vi "HVenable2.vi"(0 "Strings in":string[](array[string])=["C:\\CuspControl\\GPIB and Network\\Cusp\\Dummyfile.txt", "6723"], 1 "Dubs in":dbl[](array[numeric])=[1.0, 20.0]) -> ()   [LabVIEW 2018]
uses:
  <vilib>/DAQmx/write.llb/DAQmx Write (Analog 1D DBL NChan 1Samp).vi
  <vilib>/DAQmx/create/channels.llb/DAQmx Create Channel (AO-Voltage-Basic).vi
  <vilib>/DAQmx/miscellaneous.llb/DAQmx Fill In Error Info.vi
panel:
  in  "Gain (15 V/V)":dbl=15.0
  out "Outvolts":dbl[](array[numeric])
  in  "Enable":bool
  in  "Amplitude (V)":dbl
  in  "subvi":bool=TRUE
  out "error out":errorcluster
  in  "AO2 name":string="6723"
  in  "ao lines":string[](array[string])=["/ao5", "/ao6"]
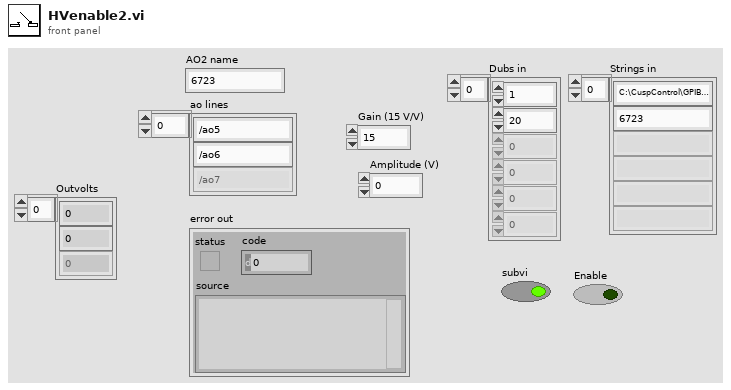
[diagram p1: front panel]
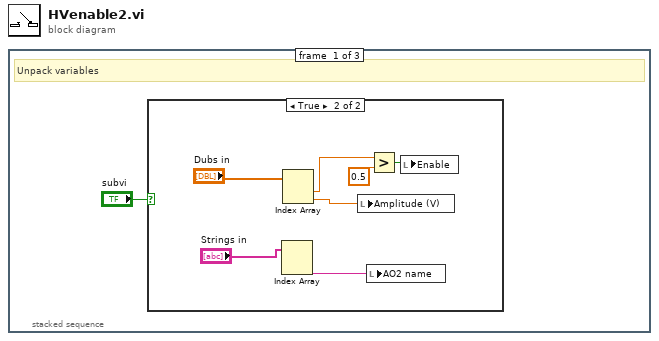
[diagram p0: block diagram]
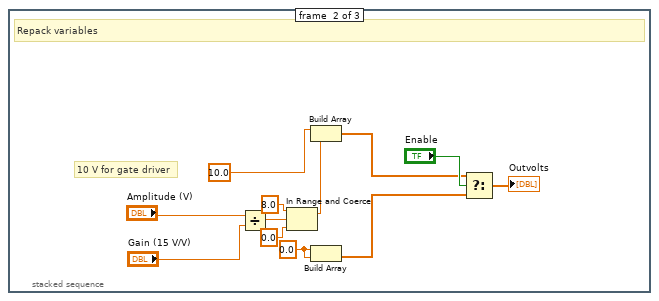
[diagram p3: hidden frame]
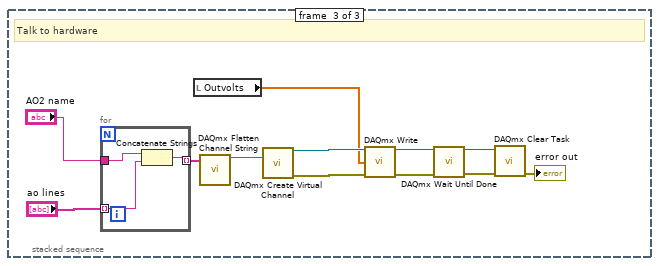
[diagram p4: hidden frame]
diagram:
  n1 = stacked-sequence {
    frame #0 {
      # "Unpack variables"
      n2 = case shown="True" "subvi" {
        frame False {
        }
        frame True {
          n3 = Index Array(array="Strings in") -> (element #2=w6:string)  [unwired: 2 in, 1 out]
          n4 = Index Array(array="Dubs in") -> (element #1=w3:dbl, element #2=w2:dbl)  [unwired: 2 in]
          n5 = local write "Amplitude (V)"(w2) -> ()
          n6 = local write "AO2 name"(w6) -> ()
          n7 = Greater?(x=w3, y=0.5) -> (0:w5:bool)
          n8 = local write "Enable"(w5) -> ()
        }
      }
    }
    frame #1 {
      w19 = 0.0 ("element")
      # "10 V for gate driver"
      # "Repack variables"
      n9 = Divide(x="Amplitude (V)", y="Gain (15 V/V)") -> (x/y=w12:dbl)
      n10 = In Range and Coerce(upper limit=8.0, x=w12, lower limit=0.0) -> (coerced(x)=w11:dbl)  [unwired: 1 out]
      n11 = Build Array(10.0 ("t"), w11) -> (w17:dbl[])
      n12 = Build Array(w19, w19) -> (w16:dbl[])
      n13 = Select(t=w17, s="Enable", f=w16) -> (s? t:f=→"Outvolts":dbl[])
    }
    frame #2 {
      # "Talk to hardware"
      n14 = for {
        tunnel: "ao lines" -> [w33] mode=indexing
        tunnel: "AO2 name" -> [w34]
        tunnel: [w35] -> w23 mode=indexing
        n15 = Concatenate Strings(w34, w33) -> (w35:string)
      }
      n16 = local read "Outvolts"() -> (w21:dbl[])
      n17 = call <vilib>:"DAQmx Flatten Channel String.vi"("names in"=w23) -> ("names out"=w22:string)  [unwired: 13 in, 1 out]
      n18 = call-poly <vilib>:"DAQmx Create Virtual Channel.vi"("physical channels"=w22) -> ("task out"=w32:refnum<k21>, "error out"=w31:errorcluster)  [unwired: 13 in]
      n19 = call-poly <vilib>:"DAQmx Write.vi"("task/channels in"=w32, "data"=w21, "error in"=w31) -> ("task out"=w28:refnum<k21>, "error out"=w27:errorcluster)  [unwired: 10 in, 1 out]
      n20 = call <vilib>:"DAQmx Wait Until Done.vi"("task/channels in"=w28, "error in"=w27) -> ("task out"=w30:refnum<k21>, "error out"=w29:errorcluster)  [unwired: 12 in]
      n21 = call <vilib>:"DAQmx Clear Task.vi"("task in"=w30, "error in"=w29) -> ("error out"=→"error out":errorcluster)  [unwired: 13 in]
    }
  }
